vi "校准窗口.vi"() -> ()   [LabVIEW 2016, in "NAQ_DO.lvlib"]
uses:
  NAQ_DO.lvlib
panel:
  in  "设置":bool
  in  "盐度":sgl=25.0
  in  "大气压力":dbl=101.35
  in  "温度校准":bool
  in  "温度标定参数":dbl=25.0
  in  "探头校准":bool
  in  "第二点校准":bool
  in  "第一点校准":bool
  in  "校准值二":dbl
  in  "校准值一":dbl
  in  "校准方式":enum16{"单点校准", "两点校准"}(ring)
  out "监测值":T1
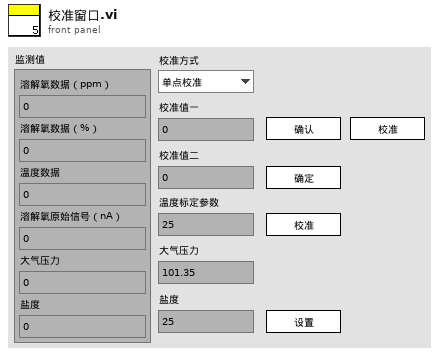
[diagram p1: front panel]
types:
  T1 = cluster{"溶解氧数据（ppm）":dbl, "溶解氧数据（%）":dbl, "温度数据":dbl, "溶解氧原始信号（nA）":dbl, "大气压力":dbl, "盐度":dbl}
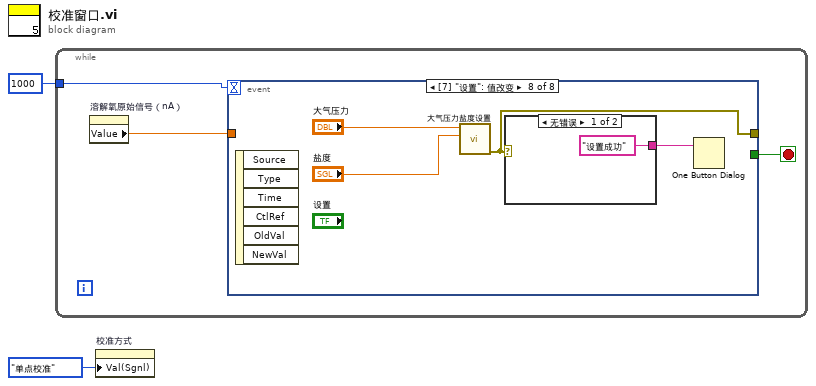
[diagram p0: block diagram]
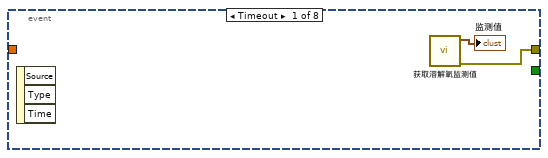
[diagram p2: hidden frame]
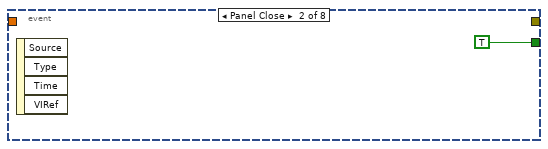
[diagram p3: hidden frame]
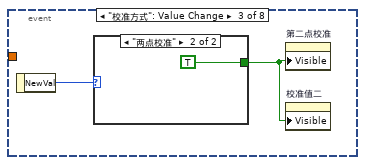
[diagram p4: hidden frame]
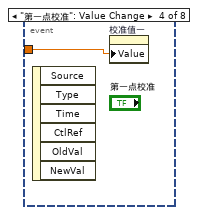
[diagram p6: hidden frame]
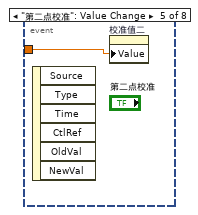
[diagram p7: hidden frame]
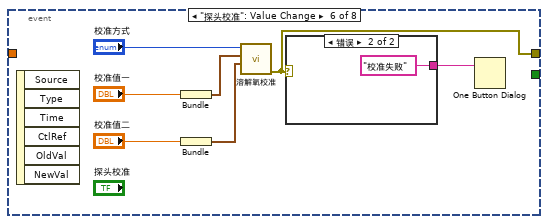
[diagram p8: hidden frame]
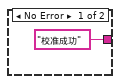
[diagram p9: hidden frame]
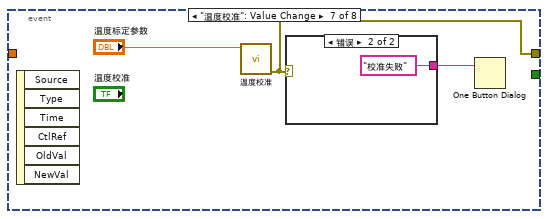
[diagram p10: hidden frame]
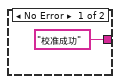
[diagram p11: hidden frame]
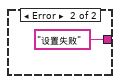
[diagram p12: hidden frame]
diagram:
  n1 = while {
    tunnel: 1000 -> [w4]
    stop <- w5 stop-if-true
    n2 = property on="溶解氧原始信号（nA）" class="DigNum (严格)"() -> ("Value"=w3:dbl)  [unwired: 2 in, 2 out]
    n3 = event shown="[7] \"设置\": 值改变" {
      selector: _ -> [_ _ _ _ _ _ _ _]
      dyn-events: _ -> [_ _ _ _ _ _ _ _]
      timeout: w4 -> [_ _ _ _ _ _ _ _]
      tunnel: [_ TRUE _ _ _ _ _ _] -> w5
      tunnel: [w6 _ _ _ _ w15 w23 w28] -> _
      tunnel: w3 -> [_ _ _ w12 w13 _ _ _]
      event Timeout {
        n4 = event-data() -> ()  [unwired: 1 in, 3 out]
        n5 = call "获取溶解氧监测值.vi"() -> ("error out"=w6:errorcluster, "监测值"=→"监测值":T1)  [unwired: 10 in]
      }
      event Panel Close {
        n6 = event-data() -> ()  [unwired: 1 in, 4 out]
      }
      event "校准方式": Value Change {
        n7 = event-data() -> ("NewVal"=w10:enum16{"单点校准", "两点校准"})  [unwired: 1 in]
        n8 = case shown="\"两点校准\"" w10 {
          tunnel: [_ TRUE] -> w9
          frame "单点校准", Default {
          }
          frame "两点校准" {
          }
        }
        n9 = property on="第二点校准" class="Bool"("Visible"=w9) -> ()  [unwired: 2 in, 2 out]
        n10 = property on="校准值二" class="DigNum (严格)"("Visible"=w9) -> ()  [unwired: 2 in, 2 out]
      }
      event "第一点校准": Value Change {
        n11 = event-data() -> ()  [unwired: 1 in, 6 out]
        n12 = property on="校准值一" class="DigNum (严格)"("Value"=w12) -> ()  [unwired: 2 in, 2 out]
      }
      event "第二点校准": Value Change {
        n13 = event-data() -> ()  [unwired: 1 in, 6 out]
        n14 = property on="校准值二" class="DigNum (严格)"("Value"=w13) -> ()  [unwired: 2 in, 2 out]
      }
      event "探头校准": Value Change {
        n15 = event-data() -> ()  [unwired: 1 in, 6 out]
        n16 = Bundle("校准值一"="校准值一") -> (w19:cluster{"校准值一":dbl})  [unwired: 1 in]
        n17 = Bundle("校准值二"="校准值二") -> (w18:cluster{"校准值二":dbl})  [unwired: 1 in]
        n18 = call "溶解氧校准.vi"("标液二"=w18, "标液一"=w19, "校准方式"="校准方式") -> ("error out"=w15:errorcluster)  [unwired: 8 in]
        n19 = case shown="错误" w15 {
          tunnel: ["校准成功" "校准失败"] -> w14
          frame No Error {
          }
          frame Error {
          }
        }
        n20 = One Button Dialog(message=w14) -> ()  [unwired: 1 in, 1 out]
      }
      event "温度校准": Value Change {
        n21 = event-data() -> ()  [unwired: 1 in, 6 out]
        n22 = call "温度校准.vi"("温度标定参数"="温度标定参数") -> ("error out"=w23:errorcluster)  [unwired: 10 in]
        n23 = case shown="错误" w23 {
          tunnel: ["校准成功" "校准失败"] -> w24
          frame No Error {
          }
          frame Error {
          }
        }
        n24 = One Button Dialog(message=w24) -> ()  [unwired: 1 in, 1 out]
      }
      event "设置": Value Change {
        n25 = event-data() -> ()  [unwired: 1 in, 6 out]
        n26 = call "大气压力盐度设置.vi"("盐度"="盐度", "大气压力"="大气压力") -> ("error out"=w28:errorcluster)  [unwired: 9 in]
        n27 = case shown="无错误" w28 {
          tunnel: ["设置成功" "设置失败"] -> w29
          frame No Error {
          }
          frame Error {
          }
        }
        n28 = One Button Dialog(message=w29) -> ()  [unwired: 1 in, 1 out]
      }
    }
  }
  n29 = property on="校准方式" class="Enum (严格)"("Val(Sgnl)"=enum16{"单点校准", "两点校准"}."单点校准" ("值(信号)")) -> ()  [unwired: 2 in, 2 out]
